vi "SP Read Array.vi"(8 "error in":errorcluster, 11 "Power Setpoint in":refnum<class "Power Setpoint.lvclass">) -> (0 "error out":errorcluster, 1 "Changed or First Call?":bool, 2 "Current Setpoint":dbl[](array[numeric]), 3 "Power Setpoint out":refnum<class "Power Setpoint.lvclass">)   [LabVIEW 2023, in "Power Setpoint.lvclass"]
uses:
  Power Setpoint.lvclass
  Parents/Setpoint/Setpoint.lvclass
  Power Setpoint.lvclass/Power Setpoint.ctl
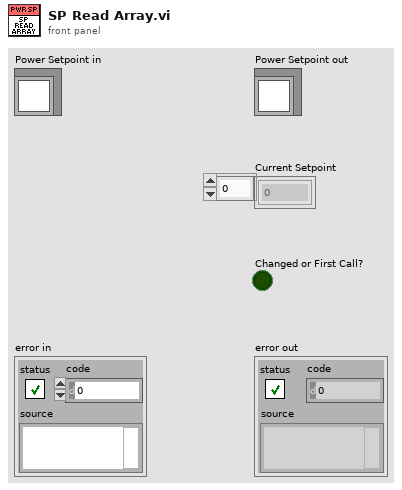
[diagram p1: front panel]
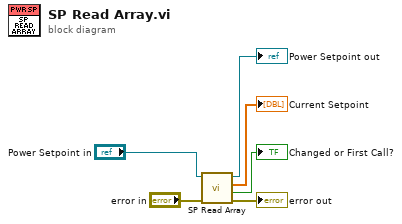
[diagram p0: block diagram]
diagram:
  n1 = call-parent "SP Read Array.vi"("error in"="error in", "Setpoint in"="Power Setpoint in") -> ("error out"=→"error out":errorcluster, "Changed or First Call?"=→"Changed or First Call?":bool, "Current Setpoint"=→"Current Setpoint":dbl[], "Setpoint out"=→"Power Setpoint out":refnum<class "Power Setpoint.lvclass">)  [unwired: 6 in]
